vi "z closure query drop.vi"(8 "error in (no error)":errorcluster, 11 "closure_":cluster{"_context":u64, "_call":u64}) -> (0 "error out":errorcluster, 3 "closure_ out":cluster{"_context":u64, "_call":u64})   [LabVIEW 2021, in "zenohc.lvlib"]
doc: "ZENOHC_API void z_closure_query_drop(struct z_moved_closure_query_t *closure_);"
uses:
  zenohc.lvlib
  zenohc.dll
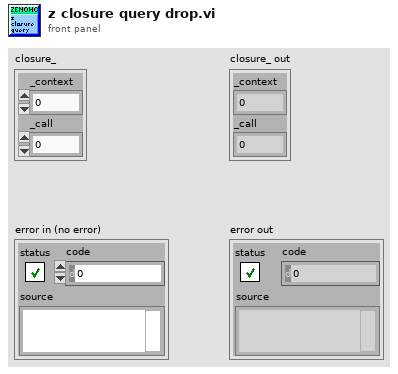
[diagram p1: front panel]
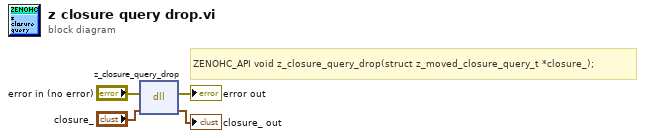
[diagram p0: block diagram]
diagram:
  # "ZENOHC_API void z_closure_query_drop(struct z_moved_closure_query_t *closure_);"
  n1 = dll-call lib="D:/dev/zenoh_labview/zenohc/zenohc.*" fn="z_closure_query_drop"(error in="error in (no error)", "closure_"="closure_") -> (error out=→"error out":errorcluster, "closure_"=→"closure_ out":cluster{"_context":u64, "_call":u64})  [unwired: 3 in, 1 out]
